vi "update_track_given_snippet.vi"(7 "Tracking Max Backwards Time (Camera Frames)":i32, 8 "Input Track":T3, 11 "Track Snippet In":T1={"Track Centroid Positions (Camera Pixel)"=[], "Within Track Index"=0, "Camera Buffer Indecies"=[], "Area (Camera Pixels)"=0, "Speed (mm/s)"=0.0, "Direction (radians)"=0.0, "Centerline Positions (Camera Pixel)"=[], "Ellipse Ratio"=0.0, "Termination Reason"=enum."StillActive", "Track Index"=-1, "Bounding Rect Left"=0, "Bounding Rect Top"=0, "Bounding Rect Right"=0, "Bounding Rect Bottom"=0, "Mature Camera Buffer"=-1, "Start Camera Buffer Index"=0, "Reverse Started Camera Buffer"=-1}) -> (0 "Output Track":T3, 3 "Track Snippet Out":T1={"Track Centroid Positions (Camera Pixel)"=[], "Within Track Index"=0, "Camera Buffer Indecies"=[], "Area (Camera Pixels)"=0, "Speed (mm/s)"=0.0, "Direction (radians)"=0.0, "Centerline Positions (Camera Pixel)"=[], "Ellipse Ratio"=0.0, "Termination Reason"=enum."StillActive", "Track Index"=-1, "Bounding Rect Left"=0, "Bounding Rect Top"=0, "Bounding Rect Right"=0, "Bounding Rect Bottom"=0, "Mature Camera Buffer"=-1, "Start Camera Buffer Index"=0, "Reverse Started Camera Buffer"=-1})   [LabVIEW 2019]
uses:
  WormTrackCluster.ctl
  StimulusObject.lvclass
  TrackTerminationReasonEnum.ctl
  WormTrackSnippetCluster.ctl
  ParametersGlobal.vi
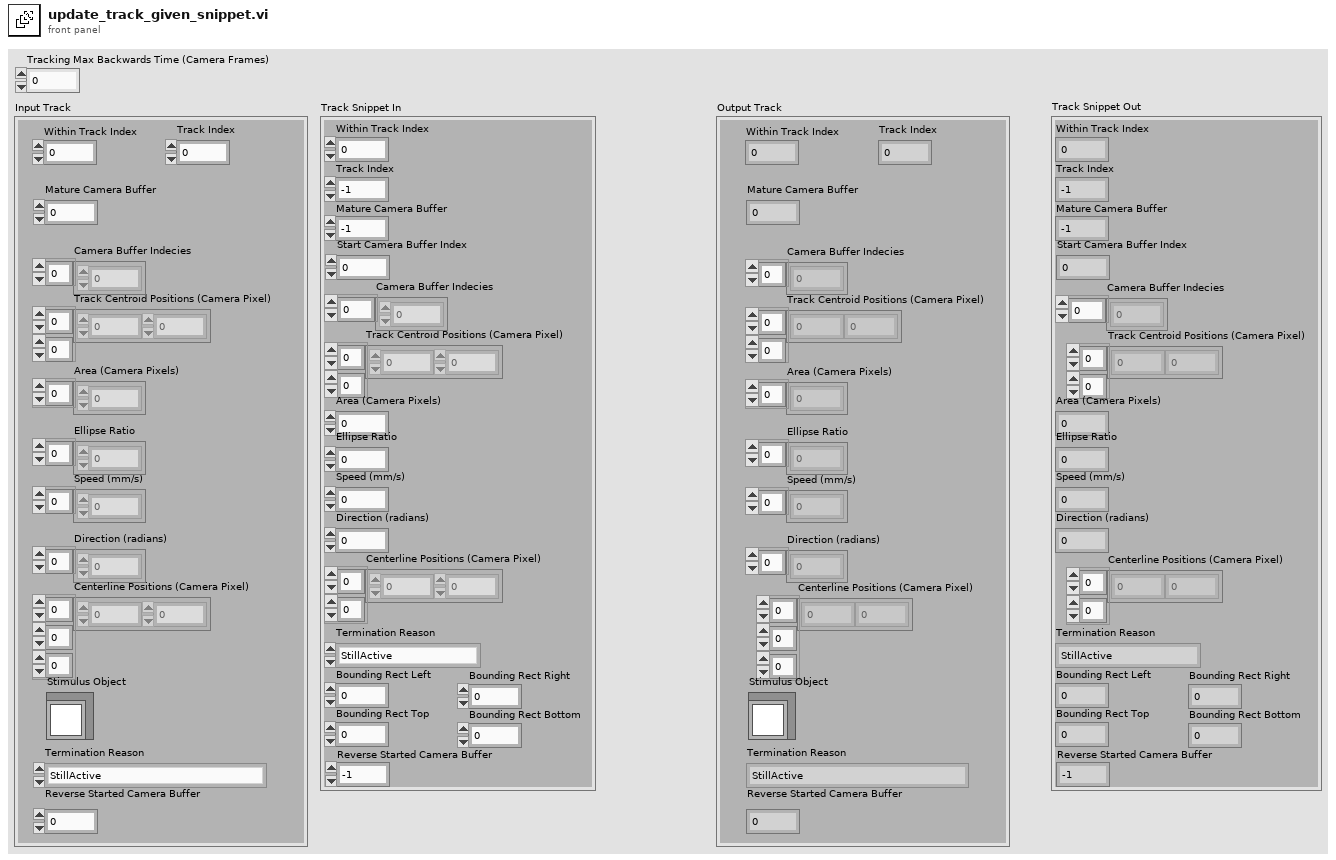
[diagram p1: front panel]
types:
  T1 = typedef "WormTrackSnippetCluster.ctl" = cluster{"Track Centroid Positions (Camera Pixel)":sgl[][], "Within Track Index":i32, "Camera Buffer Indecies":i32[], "Area (Camera Pixels)":i32, "Speed (mm/s)":sgl, "Direction (radians)":sgl, "Centerline Positions (Camera Pixel)":sgl[][], "Ellipse Ratio":sgl, "Termination Reason":T2, "Track Index":i32, "Bounding Rect Left":i32, "Bounding Rect Top":i32, "Bounding Rect Right":i32, "Bounding Rect Bottom":i32, "Mature Camera Buffer":i32, "Start Camera Buffer Index":i32, "Reverse Started Camera Buffer":i32}
  T2 = typedef "TrackTerminationReasonEnum.ctl" = enum16{"StillActive", "MaxDisplacement", "NoBlobsLeft", "AreaIncrease", "AreaDecrease", "ExperimentEnded"}
  T3 = typedef "WormTrackCluster.ctl" = cluster{"Track Centroid Positions (Camera Pixel)":sgl[][], "Within Track Index":i32, "Camera Buffer Indecies":i32[], "Area (Camera Pixels)":i32[], "Speed (mm/s)":sgl[], "Direction (radians)":sgl[], "Centerline Positions (Camera Pixel)":sgl[][][], "Ellipse Ratio":sgl[], "Stimulus Object":refnum<class "StimulusObject.lvclass">, "Termination Reason":T2, "Track Index":i32, "Mature Camera Buffer":i32, "Reverse Started Camera Buffer":i32}
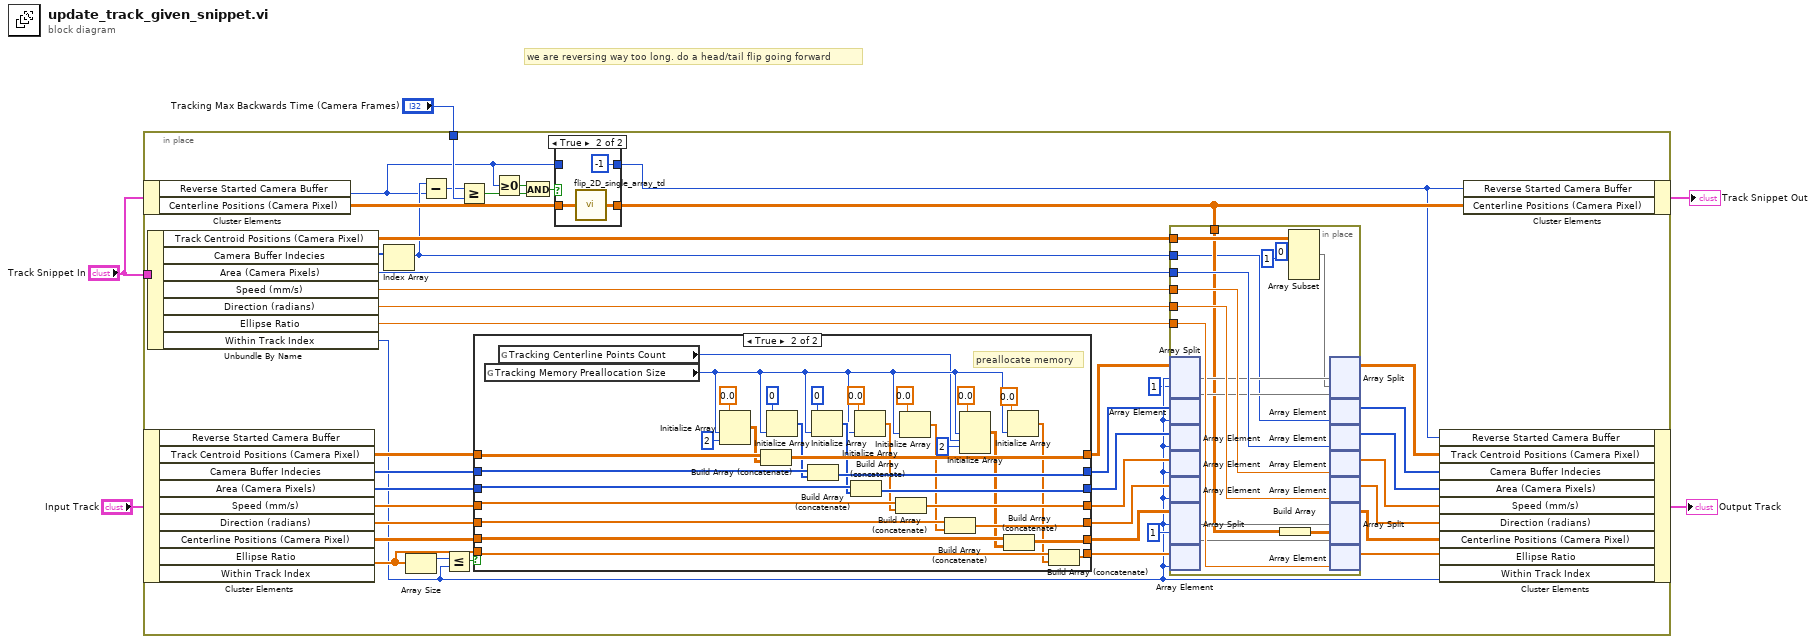
[diagram p0: block diagram]
diagram:
  # "we are reversing way too long. do a head/tail flip going forward"
  n1 = in-place {
    in-place-border: "Track Snippet In" -> [w39]
    in-place-border: "Tracking Max Backwards Time (Camera Frames)" -> [w16]
    n2 = in-place-cluster #1("Track Snippet In") -> ("Reverse Started Camera Buffer"=w9:i32, "Centerline Positions (Camera Pixel)"=w15:sgl[][])
    n3 = in-place-cluster #2("Input Track") -> ("Track Centroid Positions (Camera Pixel)"=w46:sgl[][], "Camera Buffer Indecies"=w45:i32[], "Area (Camera Pixels)"=w44:i32[], "Speed (mm/s)"=w43:sgl[], "Direction (radians)"=w42:sgl[], "Centerline Positions (Camera Pixel)"=w41:sgl[][][], "Ellipse Ratio"=w40:sgl[])  [unwired: 2 out]
    n4 = Unbundle By Name(w39) -> ("Track Centroid Positions (Camera Pixel)"=w28:sgl[][], "Camera Buffer Indecies"=w12:i32[], "Area (Camera Pixels)"=w29:i32, "Speed (mm/s)"=w30:sgl, "Direction (radians)"=w31:sgl, "Ellipse Ratio"=w37:sgl, "Within Track Index"=w21:i32)
    n5 = Index Array(array=w12) -> (element=w11:i32)  [unwired: 1 in]
    n6 = Array Size(array=w40) -> (size(s)=w48:i32)
    n7 = Subtract(x=w11, y=w9) -> (x-y=w10:i32)
    n8 = Less Or Equal?(x=w48, y=w21) -> (x <= y?=w47:bool)
    n9 = Greater Or Equal?(x=w10, y=w16) -> (x >= y?=w8:bool)
    n10 = case shown="True" w47 {
      tunnel: w40 -> [w69 w86]
      tunnel: w41 -> [w70 w88]
      tunnel: w42 -> [w71 w92]
      tunnel: w43 -> [w72 w97]
      tunnel: w44 -> [w73 w101]
      tunnel: w45 -> [w74 w105]
      tunnel: w46 -> [w75 w107]
      tunnel: [w75 w106] -> w22
      tunnel: [w74 w104] -> w23
      tunnel: [w73 w100] -> w24
      tunnel: [w72 w98] -> w26
      tunnel: [w71 w93] -> w32
      tunnel: [w70 w89] -> w36
      tunnel: [w69 w87] -> w38
      frame False {
      }
      frame True {
        # "preallocate memory"
        n11 = global read "ParametersGlobal.vi" "Tracking Memory Preallocation Size"() -> (w77:i32)
        n12 = global read "ParametersGlobal.vi" "Tracking Centerline Points Count"() -> (w76:i32)
        n13 = Initialize Array(sgl 0.0 ("element"), w77, 2 ("dimension size")) -> (w81:sgl[][])
        n14 = Build Array (concatenate)(w107, w81) -> (w106:sgl[][])
        n15 = Initialize Array(0 ("Camera Buffer Index"), w77) -> (w102:i32[])
        n16 = Build Array (concatenate)(w105, w102) -> (w104:i32[])
        n17 = Initialize Array(0 ("Camera Buffer Index"), w77) -> (w99:i32[])
        n18 = Build Array (concatenate)(w101, w99) -> (w100:i32[])
        n19 = Initialize Array(sgl 0.0 ("Camera Buffer Index"), w77) -> (w96:sgl[])
        n20 = Build Array (concatenate)(w97, w96) -> (w98:sgl[])
        n21 = Initialize Array(sgl 0.0 ("Camera Buffer Index"), w77) -> (w90:sgl[])
        n22 = Build Array (concatenate)(w92, w90) -> (w93:sgl[])
        n23 = Initialize Array(sgl 0.0 ("element"), w77, w76, 2 ("dimension size")) -> (w80:sgl[][][])
        n24 = Build Array (concatenate)(w88, w80) -> (w89:sgl[][][])
        n25 = Initialize Array(sgl 0.0 ("Camera Buffer Index"), w77) -> (w84:sgl[])
        n26 = Build Array (concatenate)(w86, w84) -> (w87:sgl[])
      }
    }
    n27 = Greater Or Equal To 0?(x=w9) -> (x >= 0?=w7:bool)
    n28 = And(x=w7, y=w8) -> (x .and. y?=w6:bool)
    n29 = case shown="True" w6 {
      tunnel: w15 -> [w50 w53]
      tunnel: [w50 w52] -> w14
      tunnel: w9 -> [w49 _]
      tunnel: [w49 -1 ("Reverse Started Camera Buffer")] -> w13
      frame False {
      }
      frame True {
        n30 = call "flip_2D_single_array_td.vi"("Centerline"=w53) -> ("Array Flipped Top Down"=w52:sgl[][])
      }
    }
    n31 = in-place {
      in-place-border: w37 -> [w68]
      in-place-border: w31 -> [w64]
      in-place-border: w30 -> [w63]
      in-place-border: w29 -> [w62]
      in-place-border: w11 -> [w54]
      in-place-border: w28 -> [w59]
      in-place-border: w14 -> [w55]
      n32 = in-place-split #3(w22, w21, 1) -> (w61:sgl[][], w60:sgl[][])  [unwired: 1 out]
      n33 = in-place-array #4(w23, w21) -> ()  [unwired: 1 out]
      n34 = in-place-array #5(w24, w21) -> ()  [unwired: 1 out]
      n35 = in-place-array #6(w26, w21) -> ()  [unwired: 1 out]
      n36 = in-place-array #7(w32, w21) -> ()  [unwired: 1 out]
      n37 = in-place-split #8(w36, w21, 1) -> (w66:sgl[][][], w67:sgl[][][])  [unwired: 1 out]
      n38 = in-place-array #9(w38, w21) -> ()  [unwired: 1 out]
      n39 = Build Array(w55) -> (w65:sgl[][][])
      n40 = Array Subset(array=w59, index (row)=0 ("index"), length (row)=1 ("length")) -> (w56:sgl[][])  [unwired: 2 in]
      n41 = in-place-split #3(w61, w56, w60) -> (w17:sgl[][])  [unwired: 2 out]
      n42 = in-place-array #4(w54) -> (w18:i32[])  [unwired: 1 out]
      n43 = in-place-array #5(w62) -> (w19:i32[])  [unwired: 1 out]
      n44 = in-place-array #6(w63) -> (w25:sgl[])  [unwired: 1 out]
      n45 = in-place-array #7(w64) -> (w27:sgl[])  [unwired: 1 out]
      n46 = in-place-split #8(w66, w65, w67) -> (w34:sgl[][][])  [unwired: 2 out]
      n47 = in-place-array #9(w68) -> (w33:sgl[])  [unwired: 1 out]
    }
    n48 = in-place-cluster #2("Reverse Started Camera Buffer"=w13, "Track Centroid Positions (Camera Pixel)"=w17, "Camera Buffer Indecies"=w18, "Area (Camera Pixels)"=w19, "Speed (mm/s)"=w25, "Direction (radians)"=w27, "Centerline Positions (Camera Pixel)"=w34, "Ellipse Ratio"=w33, "Within Track Index"=w21) -> (→"Output Track":T3)
    n49 = in-place-cluster #1("Reverse Started Camera Buffer"=w13, "Centerline Positions (Camera Pixel)"=w14) -> (→"Track Snippet Out":T1)
  }
